vi "Playback (fetching).vi"() -> ()   [LabVIEW 2018]
doc: "This VI reads records of data from the logging table in the LabVIEW.mdb database. \n\nThe table is opened with a static cursor pointing to the first record in the table. The DB Tools Move To Next/Previous Record VIs are used to navigate through the records when the Next and Previous buttons are pressed. The data is retrieved using the DB Tools Fetch Element Data VI and the arrays are converted from variants to LabVIEW arrays."
uses:
  database example subvis/Fetching - State.ctl
  <vilib>/addons/database/Recordset.llb/Rec ObjectReference.ctl
  <vilib>/addons/database/Auxilliary.llb/DB Tools Cursor Type.ctl
  <vilib>/addons/database/Connection.llb/DB Tools Open Connec (Path).vi
  <vilib>/addons/database/Connection.llb/Conn Execute.vi
  <vilib>/addons/database/Recordset.llb/Rec Get Recordset Properties (R).vi
  <vilib>/addons/database/Recordset.llb/Rec Move To Next Record (R).vi
  <vilib>/addons/database/Recordset.llb/Rec Move To Previous Record (R).vi
  <vilib>/addons/database/Recordset.llb/Rec Fetch Binary Data (R).vi
  <vilib>/addons/database/Recordset.llb/Rec Fetch Double Data (R).vi
  <vilib>/addons/database/Recordset.llb/Rec Destroy - Connection.vi
  <vilib>/addons/database/_DB Variant To Data/Database Variant To Data.xnode
  <vilib>/addons/database/NI_Database_API.lvlib
panel:
  out "record number":i32
  in  "Previous Record":bool
  in  "Next Record":bool
  in  "Stop":bool
  out "min temperature value":dbl format="%#.6g"
  out "max temperature value":dbl format="%#.6g"
  out "min pressure value":dbl format="%#.6g"
  out "max pressure value":dbl format="%#.6g"
  out "Core Temperature":dbl[](graph)
  out "Core Pressure":dbl[](graph)
  # "Overview: Demonstrates how to fetch individual records from a database for playback.\nRequirements: Database Connectivity Toolkit\nInstructions:\n1. Make sure you have already run one of the \"Database Logging\" examples.\n2. Run this VI.\n3. Click the Previous Record and Next Record buttons to fetch individual records from the database.\n4. Click Stop to stop the VI."
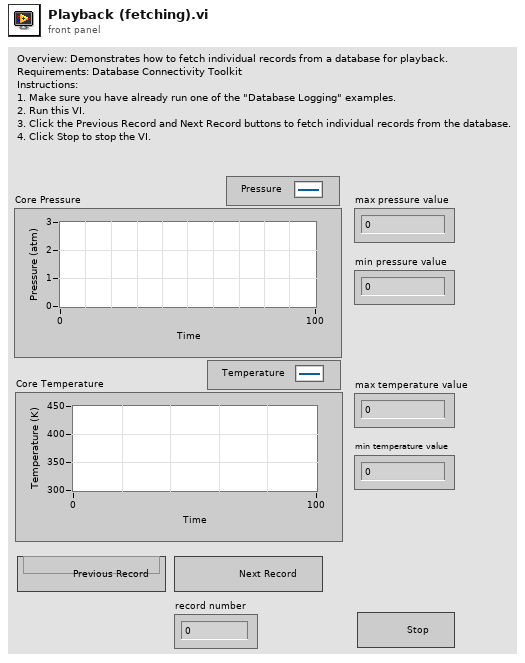
[diagram p1: front panel]
types:
  T1 = typedef "NI_Database_API.lvlib/Rec ObjectReference.ctl" = refnum<k1>
  T2 = typedef "Fetching - State.ctl" = enum16{"Initialize", "Wait for Event", "Prepare for Next", "Prepare for Previous", "Query Database", "Exit"}
  T3 = typedef "NI_Database_API.lvlib/DB Tools Cursor Type.ctl" = enum16{"forward-only", "keyset", "dynamic", "static"}
  T4 = typedef "NI_Database_API.lvlib/Conn ObjectReference.ctl" = refnum<k1>
  T5 = typedef "NI_Database_API.lvlib/Rec Properties.ctl" = cluster{"column count":i32, "record index":i32, "record count":i32, "bof?":bool, "eof?":bool, "cursor type":T3, "cache size":i32, "state":enum16{"closed", "open"}}
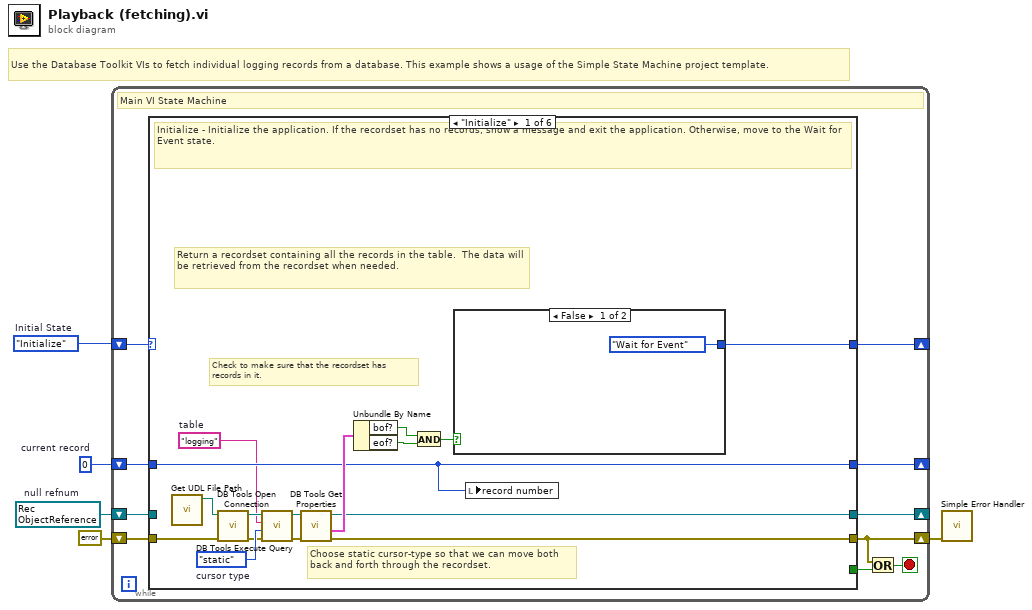
[diagram p0: block diagram]
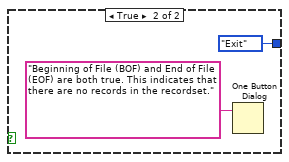
[diagram p2: hidden frame]
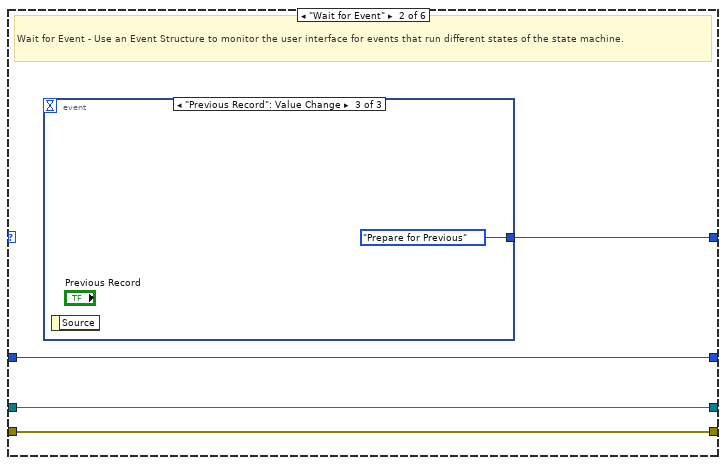
[diagram p3: hidden frame]
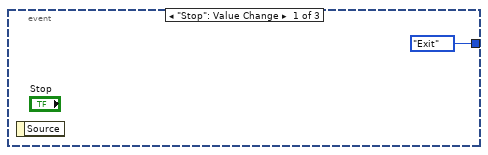
[diagram p4: hidden frame]
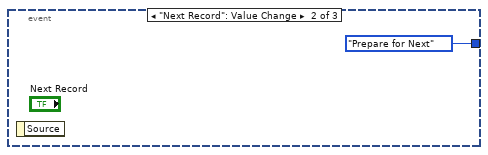
[diagram p5: hidden frame]
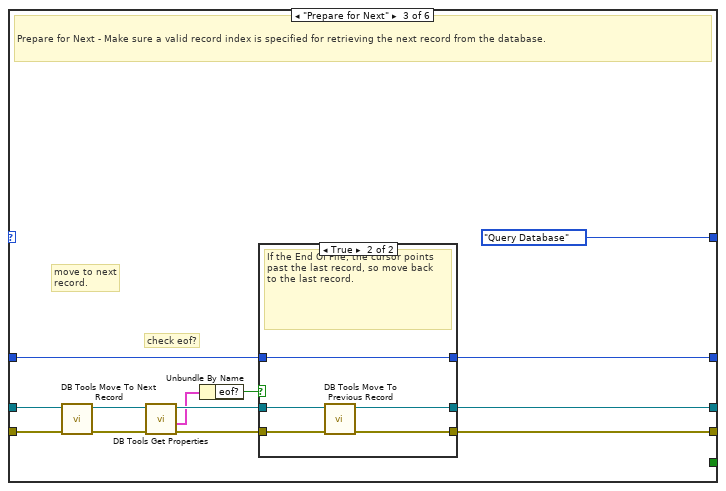
[diagram p6: hidden frame]
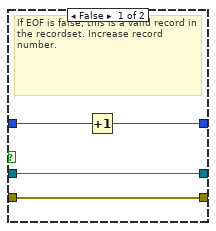
[diagram p7: hidden frame]
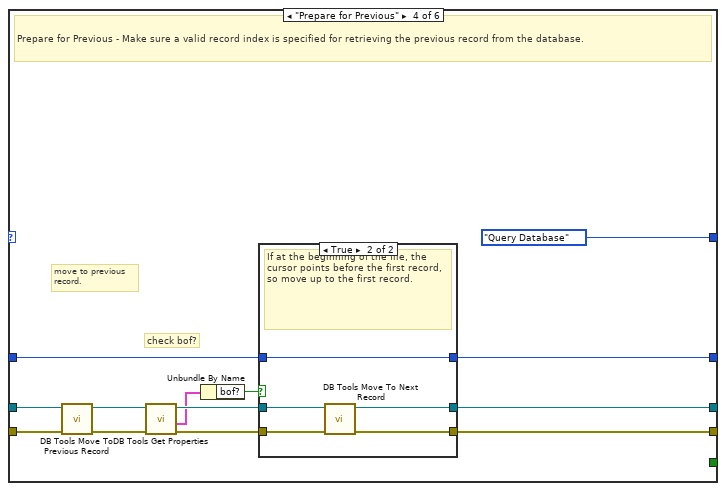
[diagram p8: hidden frame]
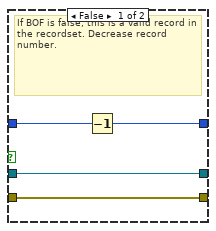
[diagram p9: hidden frame]
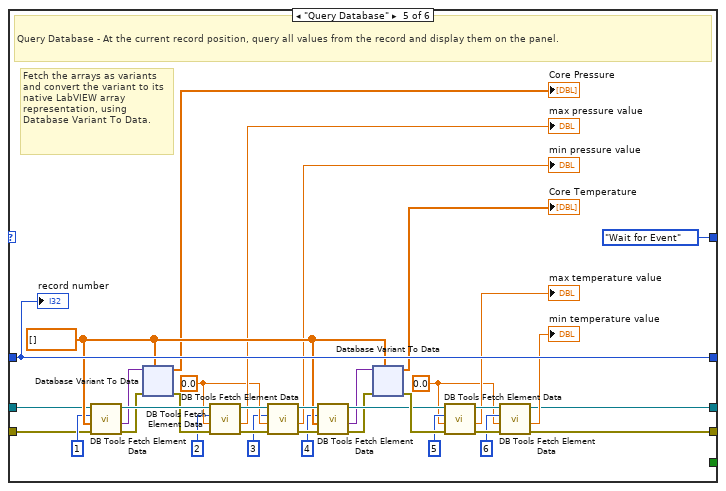
[diagram p10: hidden frame]
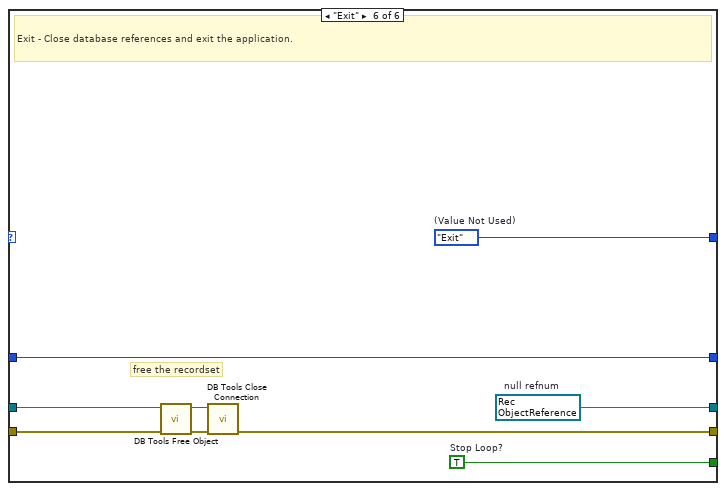
[diagram p11: hidden frame]
diagram:
  w5 = 0  # current record
  w4 = T1 refnum items=["Recordset"]  # null refnum
  w3 = Fetching_-_State."Initialize"  # Initial State
  # "Use the Database Toolkit VIs to fetch individual logging records from a database. This example shows a usage of the Simple State Machine project template."
  n1 = while {
    shift-right: [w14] -> _
    shift-left: w3 -> [w15]
    shift-right: [w10] -> w1
    shift-left: errorcluster {"status"=FALSE, "code"=0, "source"=""} ("error constant") -> [w13]
    shift-right: [w9] -> _
    shift-left: w4 -> [w8]
    shift-right: [w6] -> _
    shift-left: w5 -> [w7]
    stop <- w11 stop-if-true
    # "Main VI State Machine"
    n2 = case shown="\"Initialize\"" w15 {
      tunnel: [w18 w38 Fetching_-_State."Query Database" ("(Value Not Used)") Fetching_-_State."Query Database" ("(Value Not Used)") Fetching_-_State."Wait for Event" ("(Value Not Used)") w199] -> w14
      tunnel: [_ _ _ _ _ w198] -> w12
      tunnel: w13 -> [w22 w36 w48 w70 w90 w195]
      tunnel: [w21 w36 w47 w69 w89 w194] -> w10
      tunnel: [w20 w37 w42 w64 w87 w192] -> w9
      tunnel: w8 -> [_ w37 w43 w65 w88 w193]
      tunnel: w7 -> [w17 w35 w46 w68 w119 w191]
      tunnel: [w17 w35 w44 w66 w119 w191] -> w6
      frame "Initialize" {
        w16 = "logging"  # table
        w26 = DB_Tools_Cursor_Type."static"  # cursor type
        # "Choose static cursor-type so that we can move both back and forth through the recordset."
        # "Return a recordset containing all the records in the table.  The data will be retrieved from the recordset when needed."
        # "Check to make sure that the recordset has\nrecords in it."
        # "Initialize - Initialize the application. If the recordset has no records, show a message and exit the application. Otherwise, move to the Wait for Event state."
        n3 = call "Get UDL File Path.vi"() -> ("UDL file path"=w23:path)  [unwired: 11 in]
        n4 = call-poly <vilib>:"DB Tools Open Connection.vi"("error in (no error)"=w22, "connection information"=w23) -> ("error out"=w24:errorcluster, "connection reference"=w25:T4)  [unwired: 6 in]
        n5 = call-poly <vilib>:"DB Tools Execute Query.vi"("error in (no error)"=w24, "cursor type"=w26, "SQL query"=w16, "connection reference"=w25) -> ("error out"=w28:errorcluster, "recordset reference"=w27:T1)  [unwired: 4 in]
        n6 = call-poly <vilib>:"DB Tools Get Properties.vi"("error in (no error)"=w28, "recordset reference"=w27) -> ("error out"=w21:errorcluster, "recordset properties"=w29:T5, "recordset reference out"=w20:T1)  [unwired: 3 in]
        n7 = Unbundle By Name(w29) -> ("bof?"=w31:bool, "eof?"=w30:bool)
        n8 = And(x=w31, y=w30) -> (x .and. y?=w19:bool)
        n9 = case shown="False" w19 {
          tunnel: [Fetching_-_State."Wait for Event" ("(Value Not Used)") Fetching_-_State."Exit" ("(Value Not Used)")] -> w18
          frame False {
          }
          frame True {
            n10 = One Button Dialog(message="Beginning of File (BOF) and End of File (EOF) are both true. This indicates that there are no records in the recordset.") -> ()  [unwired: 1 in, 1 out]
          }
        }
        n11 = local write "record number"(w17) -> ()
      }
      frame "Wait for Event" {
        # "Wait for Event - Use an Event Structure to monitor the user interface for events that run different states of the state machine."
        n12 = event shown="[2] \"Previous Record\": Value Change" {
          selector: _ -> [_ _ _]
          dyn-events: _ -> [_ _ _]
          timeout: _ -> [_ _ _]
          tunnel: [Fetching_-_State."Exit" ("Next State") Fetching_-_State."Prepare for Next" ("Next State") Fetching_-_State."Prepare for Previous" ("Next State")] -> w38
          event "Stop": Value Change {
            n13 = event-data() -> ()  [unwired: 1 in, 1 out]
          }
          event "Next Record": Value Change {
            n14 = event-data() -> ()  [unwired: 1 in, 1 out]
          }
          event "Previous Record": Value Change {
            n15 = event-data() -> ()  [unwired: 1 in, 1 out]
          }
        }
      }
      frame "Prepare for Next" {
        # "check eof?"
        # "move to next\nrecord."
        # "Prepare for Next - Make sure a valid record index is specified for retrieving the next record from the database."
        n16 = call-poly <vilib>:"DB Tools Move To Next Record.vi"("error in (no error)"=w48, "recordset reference"=w43) -> ("error out"=w53:errorcluster, "recordset reference out"=w54:T1)  [unwired: 8 in]
        n17 = call-poly <vilib>:"DB Tools Get Properties.vi"("error in (no error)"=w53, "recordset reference"=w54) -> ("error out"=w52:errorcluster, "recordset properties"=w49:T5, "recordset reference out"=w51:T1)  [unwired: 3 in]
        n18 = Unbundle By Name(w49) -> ("eof?"=w50:bool)
        n19 = case shown="True" w50 {
          tunnel: w51 -> [w55 w63]
          tunnel: w52 -> [w56 w62]
          tunnel: w46 -> [w58 w61]
          tunnel: [w57 w61] -> w44
          tunnel: [w56 w60] -> w47
          tunnel: [w55 w59] -> w42
          frame False {
            # "If EOF is false, this is a valid record in the recordset. Increase record number."
            n20 = Increment(x=w58) -> (x+1=w57:i32)
          }
          frame True {
            # "If the End Of File, the cursor points\npast the last record, so move back \nto the last record."
            n21 = call-poly <vilib>:"DB Tools Move To Previous Record.vi"("error in (no error)"=w62, "recordset reference"=w63) -> ("error out"=w60:errorcluster, "recordset reference out"=w59:T1)  [unwired: 8 in]
          }
        }
      }
      frame "Prepare for Previous" {
        # "check bof?"
        # "move to previous\nrecord."
        # "Prepare for Previous - Make sure a valid record index is specified for retrieving the previous record from the database."
        n22 = call-poly <vilib>:"DB Tools Move To Previous Record.vi"("error in (no error)"=w70, "recordset reference"=w65) -> ("error out"=w75:errorcluster, "recordset reference out"=w76:T1)  [unwired: 8 in]
        n23 = call-poly <vilib>:"DB Tools Get Properties.vi"("error in (no error)"=w75, "recordset reference"=w76) -> ("error out"=w74:errorcluster, "recordset properties"=w71:T5, "recordset reference out"=w73:T1)  [unwired: 3 in]
        n24 = Unbundle By Name(w71) -> ("bof?"=w72:bool)
        n25 = case shown="True" w72 {
          tunnel: w73 -> [w77 w85]
          tunnel: w74 -> [w78 w84]
          tunnel: w68 -> [w80 w83]
          tunnel: [w79 w83] -> w66
          tunnel: [w78 w82] -> w69
          tunnel: [w77 w81] -> w64
          frame False {
            # "If BOF is false, this is a valid record in the recordset. Decrease record number."
            n26 = Decrement(x=w80) -> (x-1=w79:i32)
          }
          frame True {
            # "If at the beginning of the file, the \ncursor points before the first record, so move up to the first record."
            n27 = call-poly <vilib>:"DB Tools Move To Next Record.vi"("error in (no error)"=w84, "recordset reference"=w85) -> ("error out"=w82:errorcluster, "recordset reference out"=w81:T1)  [unwired: 8 in]
          }
        }
      }
      frame "Query Database" {
        w86 = 0.0
        w97 = 0.0
        w112 = dbl[] [] ("Array Constant")
        # "Fetch the arrays as variants and convert the variant to its native LabVIEW array representation, using Database Variant To Data."
        # "Query Database - At the current record position, query all values from the record and display them on the panel."
        n28 = call-poly <vilib>:"DB Tools Fetch Element Data.vi"("error in (no error)"=w90, "type"=w112, "column index"=1, "recordset reference"=w88) -> ("error out"=w102:errorcluster, "data"=w101:variant, "recordset reference out"=w113:T1)  [unwired: 3 in]
        n29 = xnode "Database Variant To Data"("database variant"=w101, "error in (no error)"=w102, "type"=w112) -> ("data"=→"Core Pressure":dbl[], "error out"=w100:errorcluster)
        n30 = call-poly <vilib>:"DB Tools Fetch Element Data.vi"("error in (no error)"=w100, "type"=w97, "column index"=2, "recordset reference"=w113) -> ("error out"=w115:errorcluster, "data"=→"max pressure value":dbl, "recordset reference out"=w114:T1)  [unwired: 3 in]
        n31 = call-poly <vilib>:"DB Tools Fetch Element Data.vi"("error in (no error)"=w115, "type"=w97, "column index"=3, "recordset reference"=w114) -> ("error out"=w117:errorcluster, "data"=→"min pressure value":dbl, "recordset reference out"=w116:T1)  [unwired: 3 in]
        n32 = call-poly <vilib>:"DB Tools Fetch Element Data.vi"("error in (no error)"=w117, "type"=w112, "column index"=4, "recordset reference"=w116) -> ("error out"=w107:errorcluster, "data"=w106:variant, "recordset reference out"=w110:T1)  [unwired: 3 in]
        n33 = xnode "Database Variant To Data"("database variant"=w106, "error in (no error)"=w107, "type"=w112) -> ("data"=→"Core Temperature":dbl[], "error out"=w118:errorcluster)
        n34 = call-poly <vilib>:"DB Tools Fetch Element Data.vi"("error in (no error)"=w118, "type"=w86, "column index"=5, "recordset reference"=w110) -> ("error out"=w99:errorcluster, "data"=→"max temperature value":dbl, "recordset reference out"=w111:T1)  [unwired: 3 in]
        n35 = call-poly <vilib>:"DB Tools Fetch Element Data.vi"("error in (no error)"=w99, "type"=w86, "column index"=6, "recordset reference"=w111) -> ("error out"=w89:errorcluster, "data"=→"min temperature value":dbl, "recordset reference out"=w87:T1)  [unwired: 3 in]
        "record number" <- w119
      }
      frame "Exit" {
        w192 = T1 refnum items=["Recordset"]  # null refnum
        w198 = TRUE  # Stop Loop?
        w199 = Fetching_-_State."Exit"  # (Value Not Used)
        # "free the recordset"
        # "Exit - Close database references and exit the application."
        n36 = call-poly <vilib>:"DB Tools Free Object.vi"("error in (no error)"=w195, "recordset reference"=w193) -> ("error out"=w197:errorcluster, "connection reference"=w196:T4)  [unwired: 8 in]
        n37 = call <vilib>:"DB Tools Close Connection.vi"("error in (no error)"=w197, "connection reference"=w196) -> ("error out"=w194:errorcluster)  [unwired: 5 in]
      }
    }
    n38 = Or(x=w10, y=w12) -> (x .or. y?=w11:bool)
  }
  n39 = call <vilib>:"Simple Error Handler.vi"("error in (no error)"=w1) -> ()  [unwired: 4 in, 5 out]
